vi "Initialise.vi"(8 "error in (no error)":errorcluster, 10 "Message in":refnum<class "InitialiseMessage.lvclass">, 11 "MeritFactor in":refnum<class "MeritFactor.lvclass">) -> (0 "error out":errorcluster, 3 "MeritFactor out":refnum<class "MeritFactor.lvclass">)   [LabVIEW 2012, in "MeritFactor.lvclass"]
doc: "This method is called when an initialise message is received. It mainly initialises the RabbitMQ connectivity. \n\nOverride this method when your component needs special initialisation (e.g. of software or hardware resources). In that case, don't forget to call the parent for proper implementation. If your component owns subcomponents, they count as resources, so you have to initialise them by calling their own initialise functions"
uses:
  MeritFactor.lvclass
  <vilib>/Distrio/Murmex/InitialiseMessage/InitialiseMessage.lvclass
  <vilib>/Distrio/Murmex/Murmex/Murmex.lvclass
  MeritFactor.lvclass/MeritFactor.ctl
panel:
  # "This method is called when the INTIALISE\ntrigger is sent. \n\nOverride this method when your component needs to\nrespond to this trigger. \n\nCall parent for proper implementation"
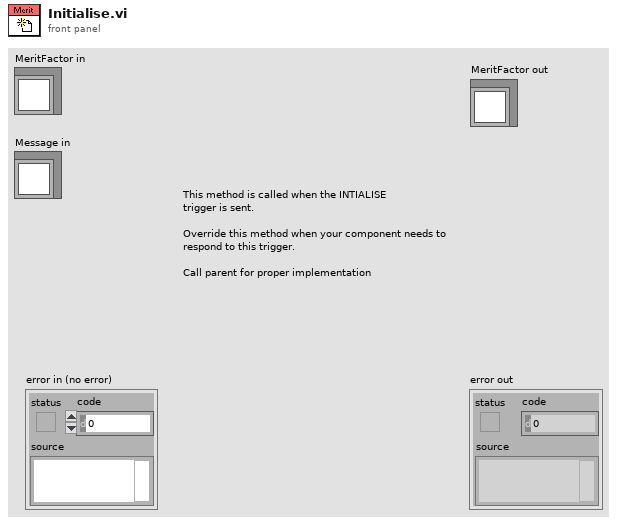
[diagram p1: front panel]
types:
  T1 = typedef "Image Type" = u32
  T2 = typedef "IMAQ Image.ctl" = refnum<image>
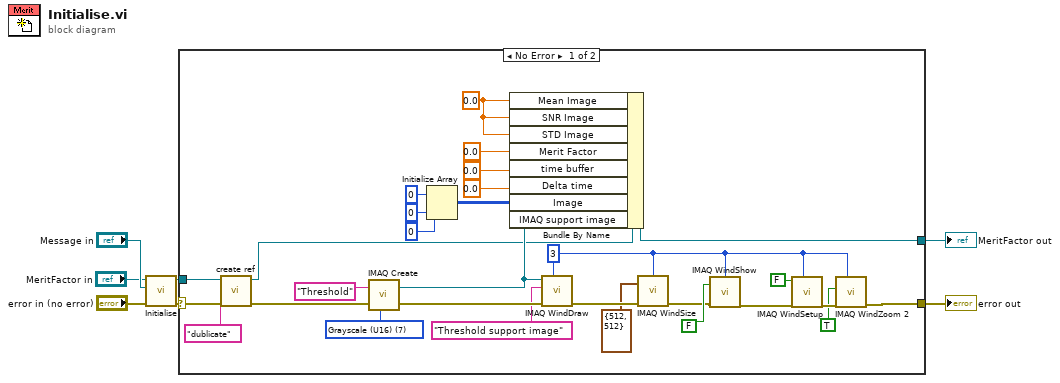
[diagram p0: block diagram]
diagram:
  n1 = call-parent "Initialise.vi"("error in (no error)"="error in (no error)", "Message in"="Message in", "Murmex in"="MeritFactor in") -> ("error out"=w4:errorcluster, "Murmex out"=w3:refnum<class "MeritFactor.lvclass">)  [unwired: 7 in]
  n2 = case shown="No Error" w4 {
    selector: w4 -> [w12 w37]
    tunnel: w3 -> [w10 w38]
    tunnel: [w29 w38] -> w2
    tunnel: [w16 w37] -> w1
    frame No Error {
      w14 = 3 ("Window Number (0...15)")
      w26 = T1 7 items=["Grayscale (U8)", "Grayscale (I16)", "Grayscale (SGL)", "Complex (CSG)", "RGB (U32)", "HSL (U32)", "RGB (U64)", "Grayscale (U16)"] ("Image Type")
      w28 = sgl 0.0 ("run-time cluster.Mean Image")
      n3 = call-dynamic "create ref.vi"("error in (no error)"=w12, "Image Name"="dublicate", "MeritFactor in"=w10) -> ("error out"=w11:errorcluster, "MeritFactor out"=w9:refnum<class "MeritFactor.lvclass">)  [unwired: 7 in]
      n4 = call "IMAQ Create"("Image Name"="Threshold", "Image Type"=w26, "error in (no error)"=w11) -> ("New Image"=w24:T2, "error out"=w25:errorcluster)  [unwired: 2 in]
      n5 = Initialize Array(u16 0 ("element"), 0 ("dimension size"), 0 ("dimension size")) -> (w36:u16[][])
      n6 = Bundle By Name(cluster=w9, "Mean Image"=w28, "SNR Image"=w28, "STD Image"=w28, "Merit Factor"=0.0 ("settings cluster.Merit Factor"), "time buffer"=0.0 ("run-time cluster.time buffer"), "Delta time"=0.0 ("run-time cluster.Delta time"), "Image"=w36, "IMAQ support image"=w24) -> (w29:refnum<class "MeritFactor.lvclass">)
      n7 = call "IMAQ WindDraw"("Window Number (0...15)"=w14, "error in (no error)"=w25, "Title"="Threshold support image", "Image"=w24) -> ("error out"=w22:errorcluster)  [unwired: 6 in, 1 out]
      n8 = call "IMAQ WindSize"("error in (no error)"=w22, "Width & Height"=cluster{"Width":i32, "Height":i32} {"Width"=512, "Height"=512}, "Window Number"=w14) -> ("error out"=w15:errorcluster)  [unwired: 3 in, 2 out]
      n9 = call "IMAQ WindShow"("error in (no error)"=w15, "Hide/Show (Show)"=FALSE, "Window Number (0...15)"=w14) -> ("error out"=w19:errorcluster)  [unwired: 3 in, 2 out]
      n10 = call "IMAQ WindSetup"("Window Number (0...15)"=w14, "error in (no error)"=w19, "Window can grow? (Yes)"=FALSE) -> ("error out"=w18:errorcluster)  [unwired: 8 in]
      n11 = call "IMAQ WindZoom 2"("Window Number (0...15)"=w14, "error in (no error)"=w18, "Zoom to Fit? (False)"=TRUE) -> ("error out"=w16:errorcluster)  [unwired: 5 in, 3 out]
    }
    frame Error {
    }
  }
  "error out" <- w1
  "MeritFactor out" <- w2
